vi "Emergency Broadcast.vi"(8 "error in (no error)":errorcluster, 10 "Message In":refnum<class "Message.lvclass">, 11 "Map Tree Queue Messenger in":refnum<class "Map Tree Queue Messenger.lvclass">) -> (0 "error out":errorcluster, 3 "Map Tree Queue Messenger out":refnum<class "Map Tree Queue Messenger.lvclass">)   [LabVIEW 2019, in "Map Tree Queue Messenger.lvclass"]
uses:
  Map Tree Queue Messenger.lvclass
  C:/Users/iio/Desktop/Bussiness/MultiSPIM/General Library/Ancestor Class/Messenger/Messenger Map Composite/Messenger Map Composite.lvclass
  Ancestor Class/Message/Message.lvclass
  Map Tree Queue Messenger.lvclass/Map Tree Queue Messenger.ctl
  Ancestor Class/Messenger/Messenger Map Composite/Messenger Map Composite.lvclass/Messenger Map Composite.ctl
  Ancestor Class/Messenger/Messenger Map Composite/Public Data/Read Child Nodes.vi
  Ancestor Class/Messenger/Messenger/Messenger.lvclass
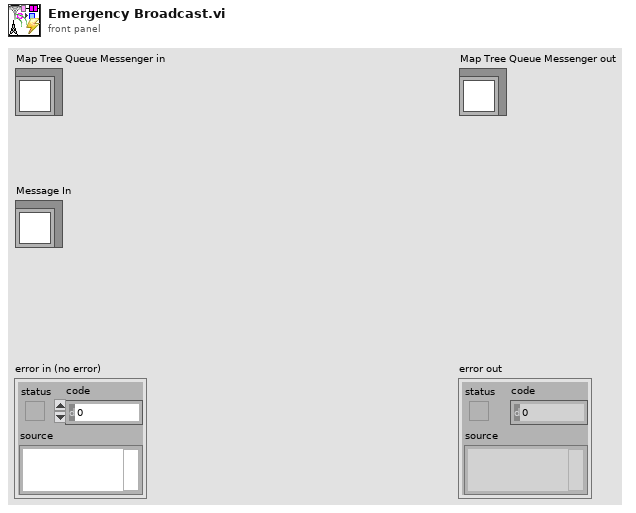
[diagram p1: front panel]
types:
  T1 = typedef "Message Queue.ctl" = refnum<queue>
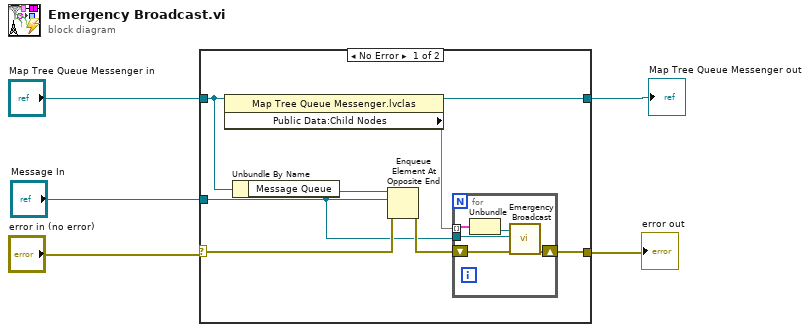
[diagram p0: block diagram]
diagram:
  n1 = case shown="No Error" "error in (no error)" {
    selector: "error in (no error)" -> [w12 w20]
    tunnel: [w10 w20] -> w1
    tunnel: [w7 w19] -> w4
    tunnel: "Map Tree Queue Messenger in" -> [w8 w19]
    tunnel: "Message In" -> [w9 _]
    frame No Error {
      n2 = property class="Map Tree Queue Messenger.lvclas"(reference=w8) -> (reference out=w7:refnum<class "Map Tree Queue Messenger.lvclass">, "Public Data:Child Nodes"=w6:map{i64, refnum<class "Messenger.lvclass">})  [unwired: 1 in, 1 out]
      n3 = Unbundle By Name(w8) -> ("Message Queue"=w13:T1)
      n4 = Enqueue Element At Opposite End(queue=w13, element=w9, error in (no error)=w12) -> (error out=w11:errorcluster)  [unwired: 1 in, 2 out]
      n5 = for {
        shift-right: [w16] -> w10
        shift-left: w11 -> [w17]
        tunnel: w6 -> [w15] mode=indexing
        tunnel: w9 -> [w18]
        n6 = Unbundle(w15) -> ("Messenger"=w14:refnum<class "Messenger.lvclass">)  [unwired: 1 out]
        n7 = call-dynamic "Emergency Broadcast.vi"("error in (no error)"=w17, "Message In"=w18, "Messenger in"=w14) -> ("error out"=w16:errorcluster)  [unwired: 7 in, 1 out]
      }
    }
    frame Error {
    }
  }
  "error out" <- w1
  "Map Tree Queue Messenger out" <- w4
